vi "4_5 Construct a VI Pro3.vi"() -> ()   [LabVIEW 2025]
panel:
  in  "stop":bool
  out "Miles":dbl
  out "Meters":dbl
  in  "Feet":dbl
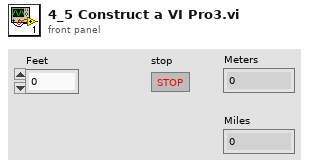
[diagram p1: front panel]
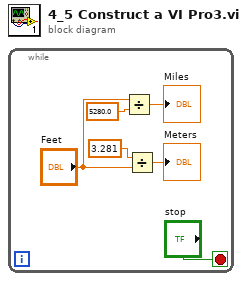
[diagram p0: block diagram]
diagram:
  n1 = while {
    stop <- "stop" stop-if-true
    n2 = Divide(x="Feet", y=5280.0) -> (x/y=→"Miles":dbl)
    n3 = Divide(x=3.281, y="Feet") -> (x/y=→"Meters":dbl)
  }
